vi "signalProcessing.vi"(9 "number of terms":i32=1, 10 "array":T1, 11 "waveform in":waveform(dbl)) -> (1 "Amplitude":dbl[](array[numeric]) format="%.2f", 2 "Frequencies":dbl[](array[numeric]) format="%.2f", 3 "output waveform":waveform(dbl))   [LabVIEW 2013]
uses:
  <vilib>/Utility/miscctls.llb/LVCursorListTypeDef.ctl
  <vilib>/Waveform/WDTOps.llb/WDT Get Waveform Subset DBL.vi
  <vilib>/addons/Time Frequency Analysis/Transform.llb/TFA Adaptive Transform (Waveform).vi
  <vilib>/addons/_Advanced Signal Processing/NI_AdvSigProcTFA.lvlib
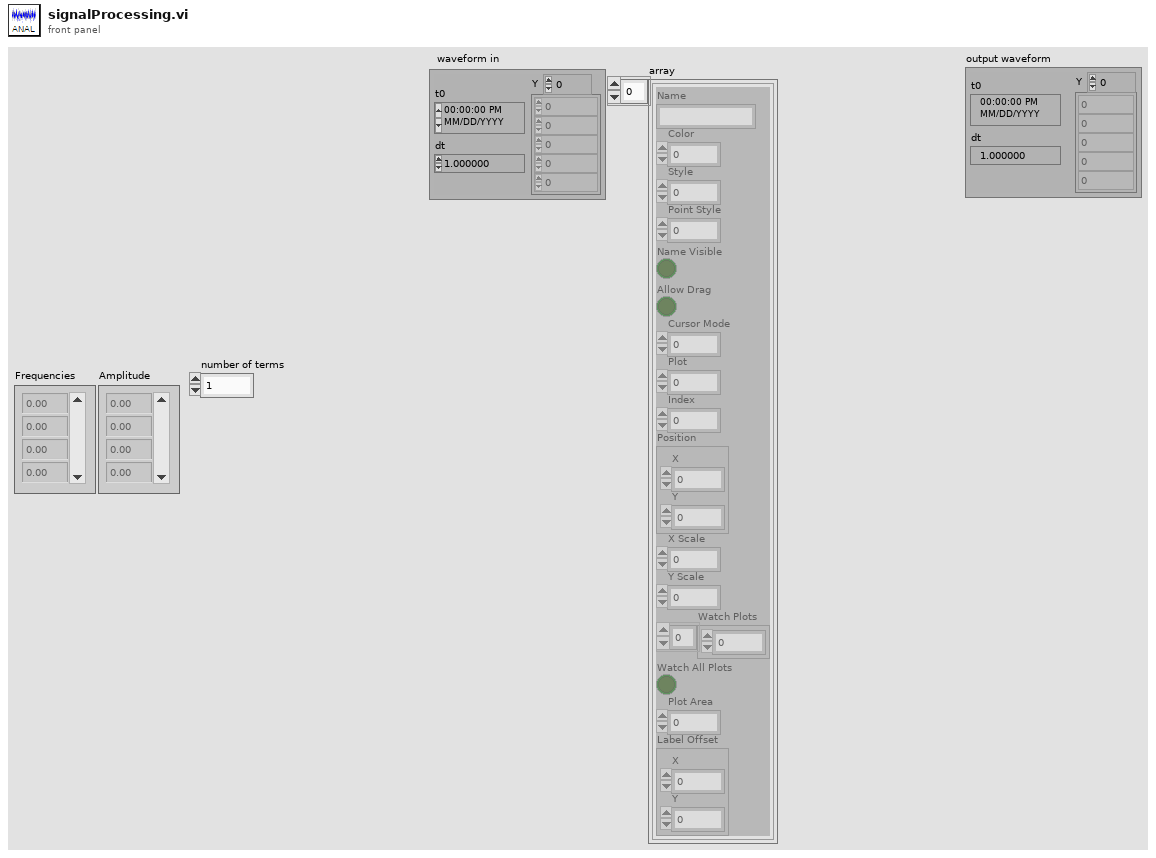
[diagram p1: front panel]
types:
  T1 = typedef "LVCursorListTypeDef.ctl" = cluster{"Name":string, "Color":u32, "Style":u8, "Point Style":u8, "Name Visible":bool, "Allow Drag":bool, "Cursor Mode":u32, "Plot":i32, "Index":i32, "Position":cluster{"X":dbl, "Y":dbl}, "X Scale":u32, "Y Scale":u32, "Watch Plots":i32[], "Watch All Plots":bool, "Plot Area":i32, "Label Offset":cluster{"X":dbl, "Y":dbl}}[]
  T2 = cluster{"Name":string, "Color":u32, "Style":u8, "Point Style":u8, "Name Visible":bool, "Allow Drag":bool, "Cursor Mode":u32, "Plot":i32, "Index":i32, "Position":cluster{"X":dbl, "Y":dbl}, "X Scale":u32, "Y Scale":u32, "Watch Plots":i32[], "Watch All Plots":bool, "Plot Area":i32, "Label Offset":cluster{"X":dbl, "Y":dbl}}
  T3 = cluster{"amplitude":cdb, "standard deviation":dbl, "center":dbl, "frequency":dbl, "chirp rate":dbl}[]
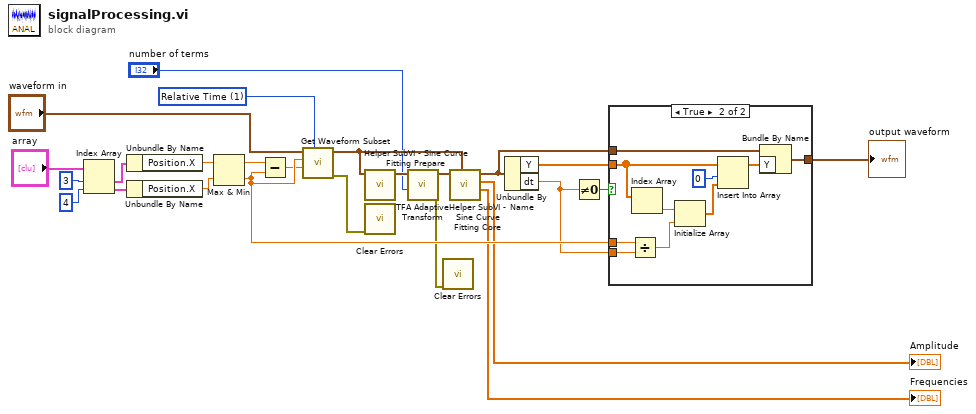
[diagram p0: block diagram]
diagram:
  w22 = u16 1 items=["Samples", "Relative Time"] ("start/duration format")
  n1 = Index Array(array="array", index #1=3 ("index"), index #2=4 ("index")) -> (element #1=w13:T2, element #2=w14:T2)
  n2 = Unbundle By Name(w13) -> ("Position.X"=w17:dbl)
  n3 = Unbundle By Name(w14) -> ("Position.X"=w18:dbl)
  n4 = Max & Min(x=w17, y=w18) -> (max(x,y)=w19:dbl, min(x,y)=w24:dbl)
  n5 = Subtract(x=w19, y=w24) -> (x-y=w20:dbl)
  n6 = call-poly <vilib>:"Get Waveform Subset.vi"("start/duration format"=w22, "duration"=w20, "start samples/time"=w24, "waveform in"="waveform in") -> ("error out"=w1:errorcluster, "waveform out"=w21:waveform(dbl))  [unwired: 2 in, 2 out]
  n7 = call "Helper SubVI - Sine Curve Fitting Prepare.vi"("signal in"=w21) -> ("signal out"=w12:waveform(dbl))  [unwired: 10 in]
  n8 = call <vilib>:"Clear Errors.vi"("error in (no error)"=w1) -> ()  [unwired: 6 in, 1 out]
  n9 = call-poly <vilib>:"TFA Adaptive Transform.vi"("number of terms"="number of terms", "signal"=w12) -> ("error out"=w2:errorcluster, "chirplet info"=w9:T3)  [unwired: 2 in, 6 out]
  n10 = call <vilib>:"Clear Errors.vi"("error in (no error)"=w2) -> ()  [unwired: 6 in, 1 out]
  n11 = call "Helper SubVI - Sine Curve Fitting Core.vi"("signal in"=w21, "ADT paras"=w9) -> ("Frequencies"=→"Frequencies":dbl[], "Amplitudes"=→"Amplitude":dbl[], "signal out"=w23:waveform(dbl))  [unwired: 7 out]
  n12 = Unbundle By Name(w23) -> ("Y"=w25:dbl[], "dt"=w3:dbl)
  n13 = Not Equal To 0?(x=w3) -> (x != 0?=w4:bool)
  n14 = case shown="True" w4 {
    tunnel: w25 -> [_ w33]
    tunnel: w3 -> [_ w29]
    tunnel: w24 -> [_ w28]
    tunnel: w23 -> [_ w27]
    tunnel: [_ w26] -> w6
    frame False {
    }
    frame True {
      n15 = Divide(x=w28, y=w29) -> (x/y=w30:dbl)
      n16 = Index Array(array=w33) -> (element=w34:dbl)  [unwired: 1 in]
      n17 = Initialize Array(w34, w30) -> (w31:dbl[])
      n18 = Insert Into Array(array=w33, index=0, new element=w31) -> (w32:dbl[])
      n19 = Bundle By Name(cluster=w27, "Y"=w32) -> (w26:waveform(dbl))
    }
  }
  "output waveform" <- w6
